vi "To XML.vi"(8 "error in (no error)":errorcluster, 9 "Parent":refnum<k20>, 10 "Document":refnum<k20>, 11 "Method in":refnum<class "Method.lvclass">) -> (0 "error out":errorcluster)   [LabVIEW 2017, in "Cobertura.lvlib" / "Method.lvclass"]
uses:
  Method.lvclass
  Method.lvclass/Method.ctl
  Line/Line.lvclass
  <resource>/objmgr/DOMUserDefRef.rc
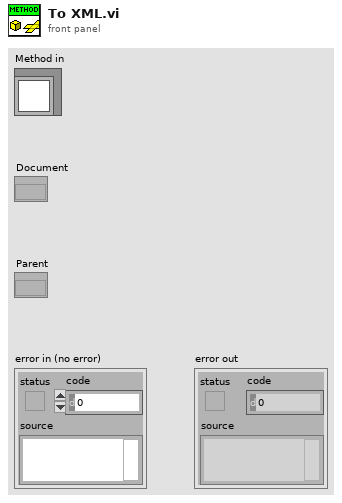
[diagram p1: front panel]
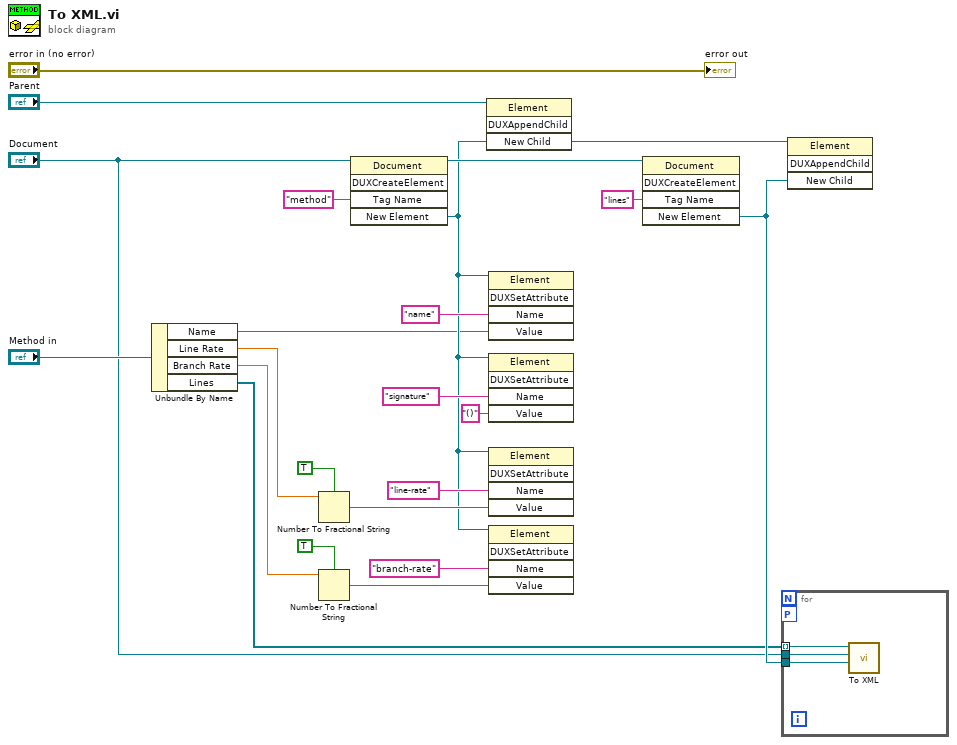
[diagram p0: block diagram]
diagram:
  n1 = Unbundle By Name("Method in") -> ("Name"=w5:string, "Line Rate"=w13:dbl, "Branch Rate"=w12:dbl, "Lines"=w1:refnum<class "Line.lvclass">[])
  n2 = Number To Fractional String(use system decimal point (T)=TRUE, number=w13) -> (F-format string=w19:string)  [unwired: 2 in]
  n3 = Number To Fractional String(use system decimal point (T)=TRUE, number=w12) -> (F-format string=w15:string)  [unwired: 2 in]
  n4 = invoke class="Document" method="DUXCreateElement"(reference="Document", "Tag Name"="method") -> (reference out=w9:refnum<k20>, "New Element"=w6:refnum<k20>)  [unwired: 3 in, 3 out]
  n5 = invoke class="Element" method="DUXAppendChild"(reference="Parent", "New Child"=w6) -> ()  [unwired: 2 in, 4 out]
  n6 = invoke class="Element" method="DUXSetAttribute"(reference=w6, "Name"="name", "Value"=w5) -> ()  [unwired: 2 in, 5 out]
  n7 = invoke class="Element" method="DUXSetAttribute"(reference=w6, "Name"="signature", "Value"="()") -> ()  [unwired: 2 in, 5 out]
  n8 = invoke class="Element" method="DUXSetAttribute"(reference=w6, "Name"="line-rate", "Value"=w19) -> ()  [unwired: 2 in, 5 out]
  n9 = invoke class="Element" method="DUXSetAttribute"(reference=w6, "Name"="branch-rate", "Value"=w15) -> ()  [unwired: 2 in, 5 out]
  n10 = invoke class="Document" method="DUXCreateElement"(reference=w9, "Tag Name"="lines") -> ("New Element"=w3:refnum<k20>)  [unwired: 3 in, 4 out]
  n11 = for {
    tunnel: w1 -> [w25] mode=indexing
    tunnel: "Document" -> [w24]
    tunnel: w3 -> [w23]
    workers-P: _ -> [_]
    n12 = call-dynamic "To XML.vi"("Parent"=w23, "Document"=w24, "Line in"=w25) -> ()  [unwired: 8 in, 1 out]
  }
  n13 = invoke class="Element" method="DUXAppendChild"(reference=w6, "New Child"=w3) -> ()  [unwired: 2 in, 4 out]
  "error out" <- "error in (no error)"
